vi "TwoSessTwoPinTwoInstrTwoSiteReservation_CallGetConnectionFromPinForOnePinAllSites_ReturnsOneConnection.vi"(8 "error in":errorcluster) -> (0 "error out":errorcluster, 2 "result":string, 3 "pass":bool)   [LabVIEW 2020, in "MeasurementServerTests.lvlib"]
uses:
  MeasurementServerTests.lvlib
  Runtime/MeasurementLink Session Management/Session Reservation/Connection.ctl
  Runtime/MeasurementLink Session Management/Session Reservation/Hardware Independent Connection.ctl
  29d31431-a3d5-4e99-b8c1-ab830a658eaa.vi
  b3e5c3be-b7a7-4b6e-86ee-709eea9cb752.vi
  29d31431-a3d5-4e99-b8c1-ab830a658eaa.vi/d089b476-b30c-4b91-b2ff-fbae0086b065.vi
  Runtime/MeasurementLink Session Management/Session Reservation/Get Connections Impl.vi
  Runtime/MeasurementLink Measurement Server/Helpers/Error Strings Global Internal.vi
  <vilib>/Utility/error.llb/Error Cluster From Error Code.vi
  Runtime/MeasurementLink Session Management/Session Reservation/Session Reservation.lvclass
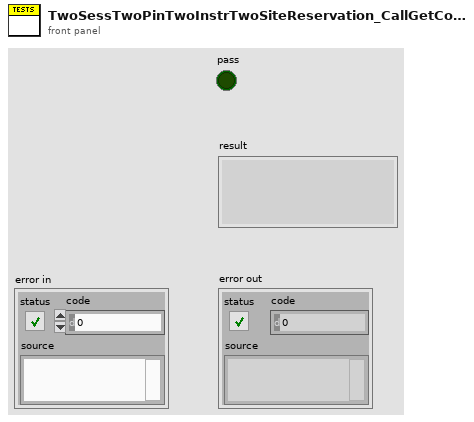
[diagram p1: front panel]
types:
  T1 = typedef "MeasurementLink Session Management.lvlib/Session Reservation.lvclass/Connection.ctl" = cluster{"connection":T2, "session":variant}
  T2 = typedef "MeasurementLink Session Management.lvlib/Session Reservation.lvclass/Hardware Independent Connection.ctl" = cluster{"pin or relay name":string, "site":i32, "instrument type id":string, "channel":string}
  T3 = typedef "MeasurementLink Session Management.lvlib/Session Reservation.lvclass/Data.ctl" = cluster{"session and driver infos":T4[], "pins":string[]}
  T4 = typedef "MeasurementLink Session Management.lvlib/Session Reservation.lvclass/Session and Driver Info.ctl" = cluster{"session info":T5, "session created":bool, "session":variant}
  T5 = typedef "MeasurementLink Session Management Client.lvlib/ni_measurementlink_sessionmanagement_v1_SessionInformation.ctl" = cluster{"session":T6, "resource_name":string, "channel_list":string, "instrument_type_id":string, "session_exists":bool, "channel_mappings":T7[]}
  T6 = typedef "MeasurementLink Session Management Client.lvlib/nidevice_grpc_Session.ctl" = cluster{"name":string}
  T7 = typedef "MeasurementLink Session Management Client.lvlib/ni_measurementlink_sessionmanagement_v1_ChannelMapping.ctl" = cluster{"pin_or_relay_name":string, "site":i32, "channel":string}
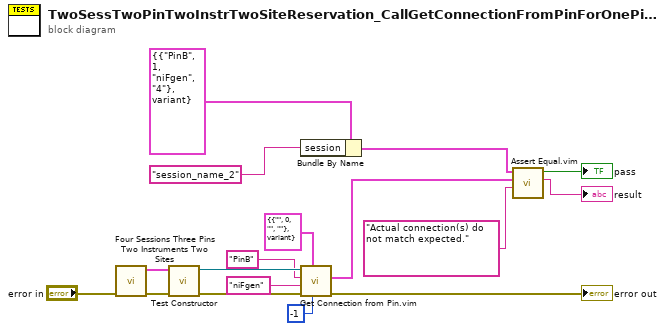
[diagram p0: block diagram]
diagram:
  n1 = call "Four Sessions Three Pins Two Instruments Two Sites.vi"("error in"="error in") -> ("error out"=w8:errorcluster, "data out"=w1:T3)  [unwired: 9 in]
  n2 = call "Test Constructor.vi"("error in"=w8, "data"=w1) -> ("error out"=w16:errorcluster, "Session Reservation out"=w15:refnum<class "Session Reservation.lvclass">)  [unwired: 8 in]
  n3 = Bundle By Name(cluster=T1 {"connection"={"pin or relay name"="PinB", "site"=1, "instrument type id"="niFgen", "channel"="4"}, "session"=variant} ("connection type"), "session"="session_name_2") -> (w2:T1)
  n4 = call "Get Connection from Pin.vim"("site"=-1, "connection type"=T1 {"connection"={"pin or relay name"="", "site"=0, "instrument type id"="", "channel"=""}, "session"=variant} ("connection"), "error in"=w16, "instrument type id"="niFgen", "pin or relay name"="PinB", "session reservation in"=w15) -> ("error out"=→"error out":errorcluster, "connection"=w12:T1)  [unwired: 3 in, 1 out]
  n5 = call "Assert Equal.vim"("failure message"="Actual connection(s) do not match expected.", "actual value"=w12, "expected value"=w2) -> ("message"=→"result":string, "equal?"=→"pass":bool)  [unwired: 7 in]
